vi "Interface_Dispatch_Get Parameter Control Refs.vi"(8 "error in (no error)":errorcluster, 11 "Dispatch_SOC Control in":refnum<class "Dispatch_SOC Control.lvclass">) -> (0 "error out":errorcluster, 1 "Dependencies Controls[]":refnum<vi>[](array[refnum]), 2 "Configuration Controls[]":refnum<vi>[](array[refnum]), 3 "Dispatch_SOC Control out":refnum<class "Dispatch_SOC Control.lvclass">, 4 "Output Controls[]":refnum<vi>[](array[refnum]))   [LabVIEW 2015, in "Dispatch_SOC Control.lvclass"]
uses:
  Dispatch_SOC Control.lvclass
  Dispatch_SOC Control_Configuration.ctl
  Dispatch_SOC Control_Dependencies.ctl
  Dispatch_SOC Control_Output.ctl
  Dispatch_SOC Control.lvclass/Dispatch_SOC Control.ctl
panel:
  out "Output":T1
  out "Dependencies":T2
  out "Configuration":T3
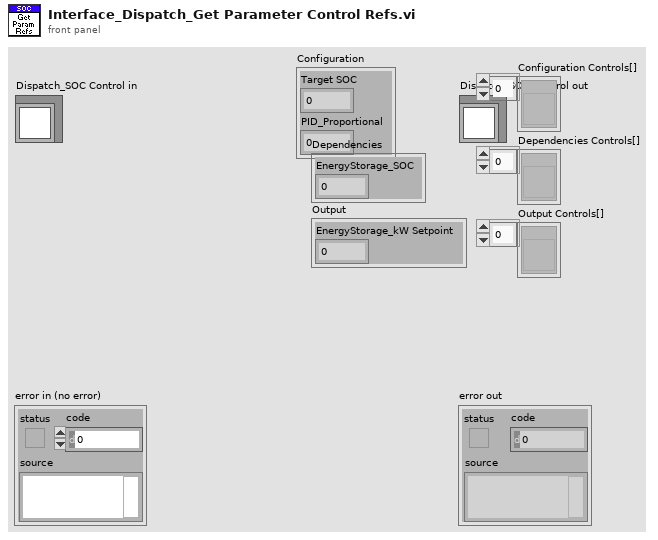
[diagram p1: front panel]
types:
  T1 = typedef "Dispatch_SOC Control.lvclass/Dispatch_SOC Control_Output.ctl" = cluster{"EnergyStorage_kW Setpoint":dbl}
  T2 = typedef "Dispatch_SOC Control.lvclass/Dispatch_SOC Control_Dependencies.ctl" = cluster{"EnergyStorage_SOC":dbl}
  T3 = typedef "Dispatch_SOC Control.lvclass/Dispatch_SOC Control_Configuration.ctl" = cluster{"Target SOC":dbl, "PID_Proportional":dbl}
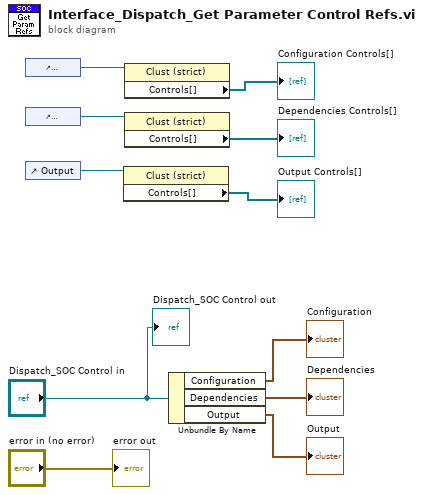
[diagram p0: block diagram]
diagram:
  n1 = control-ref of="Configuration"() -> (w5:refnum<vi>)
  n2 = control-ref of="Dependencies"() -> (w4:refnum<vi>)
  n3 = control-ref of="Output"() -> (w3:refnum<vi>)
  n4 = property class="Clust (strict)"(reference=w3) -> ("Controls[]"=→"Output Controls[]":refnum<vi>[])  [unwired: 1 in, 2 out]
  n5 = property class="Clust (strict)"(reference=w5) -> ("Controls[]"=→"Configuration Controls[]":refnum<vi>[])  [unwired: 1 in, 2 out]
  n6 = property class="Clust (strict)"(reference=w4) -> ("Controls[]"=→"Dependencies Controls[]":refnum<vi>[])  [unwired: 1 in, 2 out]
  n7 = Unbundle By Name("Dispatch_SOC Control in") -> ("Configuration"=→"Configuration":T3, "Dependencies"=→"Dependencies":T2, "Output"=→"Output":T1)
  "error out" <- "error in (no error)"
  "Dispatch_SOC Control out" <- "Dispatch_SOC Control in"
